vi "WriteConfig.vi"(8 "error in (no error)":errorcluster, 10 "Config":variant, 11 "C37.118 PMU in":refnum<class "C37.118 PMU.lvclass">) -> (0 "error out":errorcluster, 3 "C37.118 PMU out":refnum<class "C37.118 PMU.lvclass">)   [LabVIEW 2014, in "SensorPlugins.lvlib" / "C37.118 PMU.lvclass"]
uses:
  C37.118 PMU.lvclass
  PmuBaseClass/PmuBase.lvclass
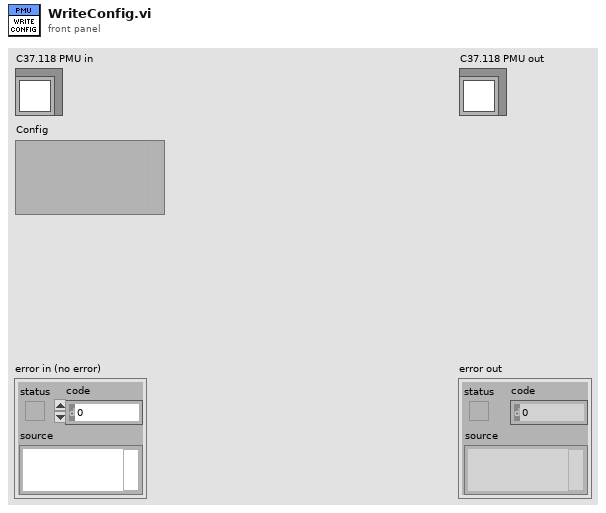
[diagram p1: front panel]
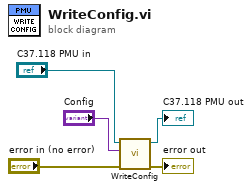
[diagram p0: block diagram]
diagram:
  n1 = call-parent "WriteConfig.vi"("error in (no error)"="error in (no error)", "Config"="Config", "PmuBase in"="C37.118 PMU in") -> ("error out"=→"error out":errorcluster, "PmuBase out"=→"C37.118 PMU out":refnum<class "C37.118 PMU.lvclass">)  [unwired: 7 in]
